vi "ShooterPneumatic.vi"(7 "Action":T1=enum."Shoot", 8 "error in":errorcluster) -> (0 "error out":errorcluster)   [LabVIEW 2013]
doc: "Shooter is used to interact ONLY with the shooter pneumatics (kicker and firing cylinder). It can be used on its own or inside CheckedShooter.vi. It has the following actions:\n-Init: takes a single solenoid reference for the kicker and firing cylinder and passes them onto the single solenoid VI.\n-Shoot:\n +Actuates the firing cylinders.\n +Waits a specified amount of time (Wait1).\n +Actuates the kicker.\n +Waits a specified amount of time (Wait2).\n +Retracts the kicker.\n +Waits a specified amount of time (Wait3).\n +Retracts the firing cylinders."
uses:
  ShooterAction.ctl
  SingleSolenoidAction.ctl
panel:
  in  "Wait3":u32
  in  "Wait2":u32=250
  in  "Wait1":u32=750
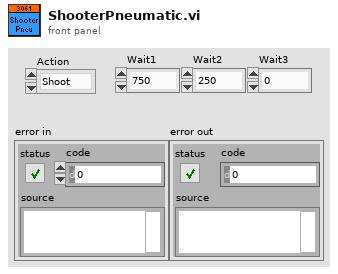
[diagram p1: front panel]
types:
  T1 = typedef "ShooterAction.ctl" = enum16{"Init", "Shoot"}
  T2 = typedef "SingleSolenoidAction.ctl" = enum16{"Init", "SetState", "Disable"}
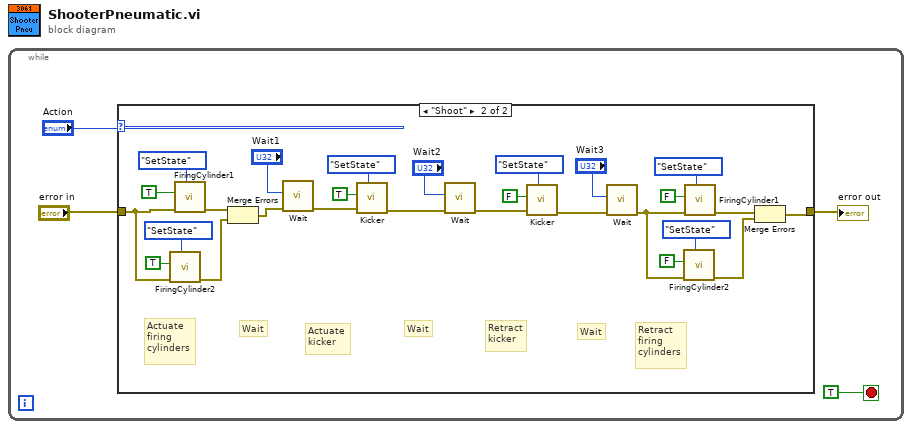
[diagram p0: block diagram]
diagram:
  n1 = while {
    stop <- TRUE stop-if-true
    n2 = case shown="\"Shoot\"" "Action" {
      tunnel: "error in" -> [w5 w16]
      tunnel: [w5 w8] -> w1
      frame "Init", Default {
        # "We shouldn't need to do anything here..."
      }
      frame "Shoot" {
        # "Retract\nfiring\ncylinders"
        # "Wait"
        # "Retract\nkicker"
        # "Wait"
        # "Actuate\nkicker"
        # "Wait"
        # "Actuate\nfiring\ncylinders"
        n3 = call "FiringCylinder2.vi"("Action"=SingleSolenoidAction."SetState", "error in (no error)"=w16, "Actuate?"=TRUE) -> ("error out"=w13:errorcluster)  [unwired: 8 in]
        n4 = call "FiringCylinder1.vi"("Action"=SingleSolenoidAction."SetState" ("Mode"), "error in (no error)"=w16, "Actuate?"=TRUE ("State")) -> ("error out"=w14:errorcluster)  [unwired: 8 in]
        n5 = Merge Errors(w14, w13) -> (w12:errorcluster)
        n6 = call "Wait.vi"("error in"=w12, "milliseconds to wait"="Wait1") -> ("error out"=w32:errorcluster)  [unwired: 9 in]
        n7 = call "Kicker.vi"("Action"=SingleSolenoidAction."SetState" ("Mode"), "error in (no error)"=w32, "Actuate?"=TRUE ("State")) -> ("error out"=w31:errorcluster)  [unwired: 8 in]
        n8 = call "Wait.vi"("error in"=w31, "milliseconds to wait"="Wait2") -> ("error out"=w30:errorcluster)  [unwired: 9 in]
        n9 = call "Kicker.vi"("Action"=SingleSolenoidAction."SetState" ("Mode"), "error in (no error)"=w30, "Actuate?"=FALSE ("State")) -> ("error out"=w29:errorcluster)  [unwired: 8 in]
        n10 = call "Wait.vi"("error in"=w29, "milliseconds to wait"="Wait3") -> ("error out"=w9:errorcluster)  [unwired: 9 in]
        n11 = call "FiringCylinder2.vi"("Action"=SingleSolenoidAction."SetState", "error in (no error)"=w9, "Actuate?"=FALSE) -> ("error out"=w6:errorcluster)  [unwired: 8 in]
        n12 = call "FiringCylinder1.vi"("Action"=SingleSolenoidAction."SetState" ("Mode"), "error in (no error)"=w9, "Actuate?"=FALSE ("State")) -> ("error out"=w7:errorcluster)  [unwired: 8 in]
        n13 = Merge Errors(w7, w6) -> (w8:errorcluster)
      }
    }
    "error out" <- w1
  }
